vi "NewProductDialog.vi"(8 "error in (no error)":errorcluster) -> (0 "error out":errorcluster, 1 "Cancelled?":bool, 3 "New Product":T1)   [LabVIEW 2020]
doc: "This VI generates data of New Product.\nCancelled? - indicator equals true if operation was cancelled.s"
uses:
  #typedef_Product.ctl
panel:
  in  "Cancel Button":bool
  in  "OK Button":bool
  in  "Product":T1
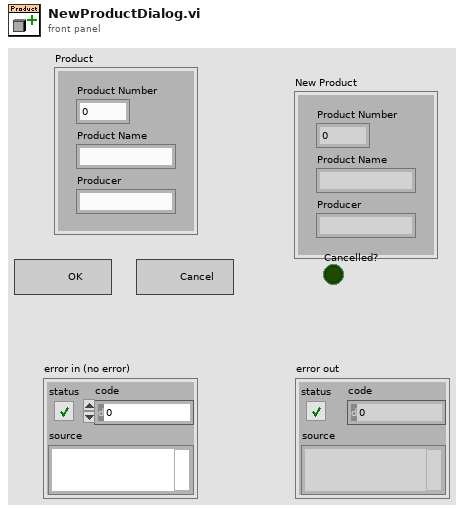
[diagram p1: front panel]
types:
  T1 = typedef "#typedef_Product.ctl" = cluster{"Product Number":i32, "Product Name":string, "Producer":string}
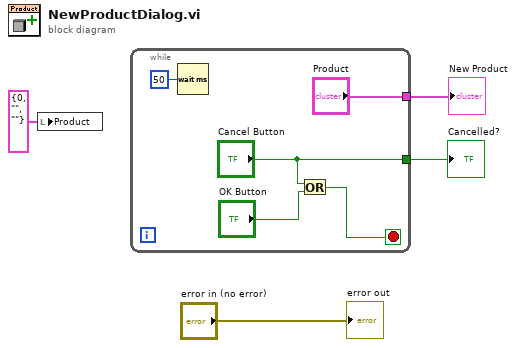
[diagram p0: block diagram]
diagram:
  n1 = local write "Product"(T1 {"Product Number"=0, "Product Name"="", "Producer"=""} ("Product")) -> ()
  n2 = while {
    tunnel: ["Product"] -> w4
    tunnel: ["Cancel Button"] -> w3
    stop <- w8 stop-if-true
    n3 = Wait (ms)(milliseconds to wait=u32 50) -> ()  [unwired: 1 out]
    n4 = Or(x="Cancel Button", y="OK Button") -> (x .or. y?=w8:bool)
  }
  "New Product" <- w4
  "Cancelled?" <- w3
  "error out" <- "error in (no error)"
